vi "Read Card Cluster Ref.vi"(8 "error in (no error)":errorcluster, 11 "Universal Power Meter in":refnum<class "Universal Power Meter.lvclass">) -> (0 "error out":errorcluster, 2 "Card Cluster Ref":refnum<vi>, 3 "Universal Power Meter out":refnum<class "Universal Power Meter.lvclass">)   [LabVIEW 2012]
uses:
  Universal Power Meter.lvclass
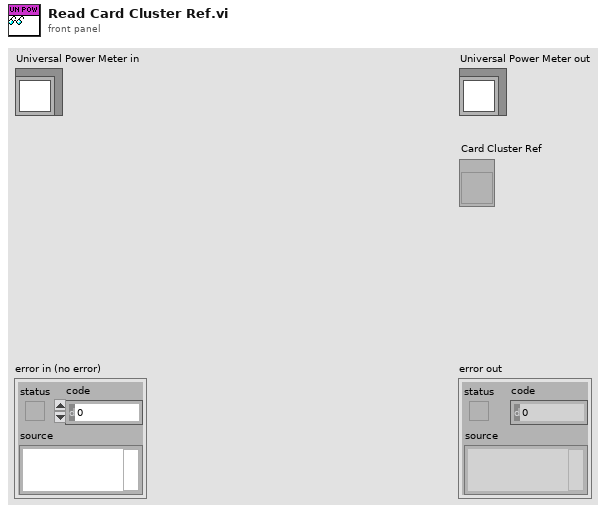
[diagram p1: front panel]
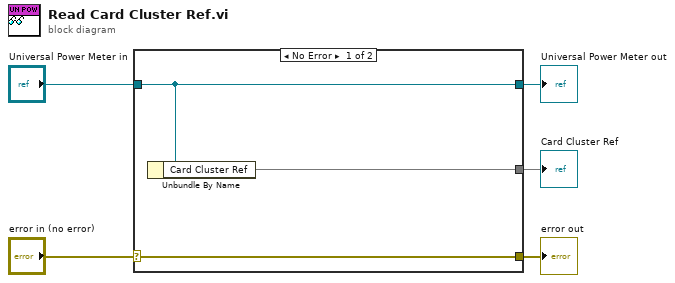
[diagram p0: block diagram]
diagram:
  n1 = case shown="No Error" "error in (no error)" {
    selector: "error in (no error)" -> [w8 w9]
    tunnel: [w8 w9] -> w4
    tunnel: [w7 w10] -> w2
    tunnel: "Universal Power Meter in" -> [w7 w10]
    tunnel: [w6 _] -> w1
    frame No Error {
      n2 = Unbundle By Name(w7) -> ("Card Cluster Ref"=w6)
    }
    frame Error {
    }
  }
  "error out" <- w4
  "Universal Power Meter out" <- w2
  "Card Cluster Ref" <- w1
